vi "MasterEnable.vi"(8 "error in (no error)":errorcluster, 10 "Master Enable":bool=TRUE, 11 "PowerSupply in":refnum<class "PowerSupply.lvclass">) -> (0 "error out":errorcluster, 3 "PowerSupply out":refnum<class "PowerSupply.lvclass">)   [LabVIEW 2020, in "PowerSupply.lvclass"]
doc: "Toggle user control all Power Supply channels."
uses:
  PowerSupply.lvclass
  C:/Code Projects/CircuitExplorer/AnalogDiscoveryFunction/AnalogDiscoveryFunction.lvclass
  AnalogDiscoveryFunction/AnalogDiscoveryFunction.lvclass/AnalogDiscoveryFunction.ctl
  AnalogDiscoveryFunction/GetInstrumentHandle.vi
  <vilib>/DigilentWF/DigilentWF.lvlib
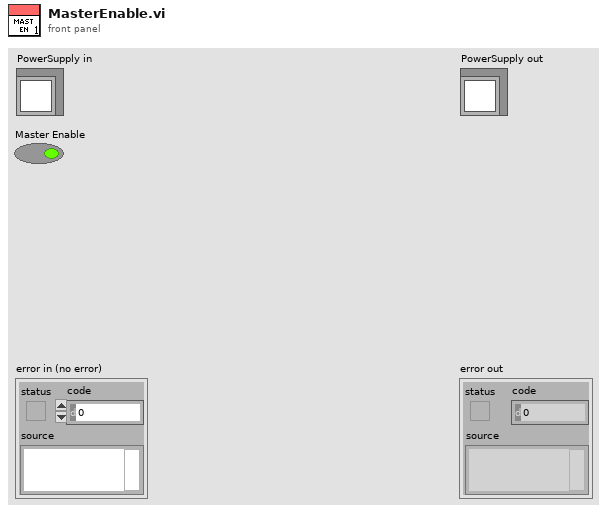
[diagram p1: front panel]
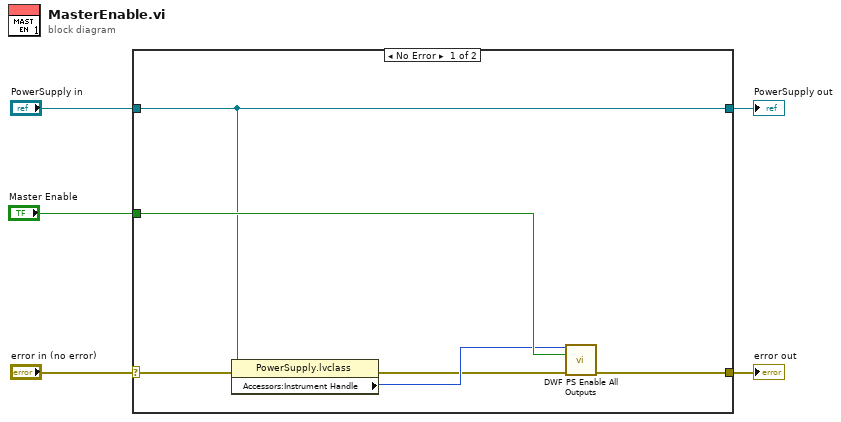
[diagram p0: block diagram]
diagram:
  n1 = case shown="No Error" "error in (no error)" {
    selector: "error in (no error)" -> [w9 w13]
    tunnel: [w10 w13] -> w4
    tunnel: [w8 w12] -> w2
    tunnel: "PowerSupply in" -> [w8 w12]
    tunnel: "Master Enable" -> [w11 _]
    frame No Error {
      n2 = property class="PowerSupply.lvclass"(reference=w8, error in=w9) -> (error out=w6:errorcluster, "Accessors:Instrument Handle"=w7:u32)  [unwired: 1 out]
      n3 = call <vilib>:"DWF PS Enable All Outputs.vi"("Instrument Handle In"=w7, "Enable Outputs"=w11, "Error In"=w6) -> ("Error Out"=w10:errorcluster)  [unwired: 11 in, 1 out]
    }
    frame Error {
    }
  }
  "error out" <- w4
  "PowerSupply out" <- w2
